vi "Homework 1.vi"() -> ()   [LabVIEW 2018]
uses:
  Control 1.ctl
  <vilib>/DAQmx/write.llb/DAQmx Write (Digital Bool 1Line 1Point).vi
  <vilib>/DAQmx/read.llb/DAQmx Read (Analog DBL 1Chan 1Samp).vi
  <vilib>/DAQmx/create/channels.llb/DAQmx Create Channel (DO-Digital Output).vi
  <vilib>/DAQmx/miscellaneous.llb/DAQmx Fill In Error Info.vi
  <vilib>/DAQmx/create/channels.llb/DAQmx Create Channel (AI-Voltage-Basic).vi
panel:
  out "Image Out":T1(plugin-control)
  in  "Izbor predmeta":enum16{"Predmet A", "Predmet B", "Predmet C"}(ring)
  in  "a":bool
  in  "Promeni predmet":bool
  in  "Ukloni alarm":bool
  in  "Pokreni traku":bool
  in  "Predmet je na traci":bool
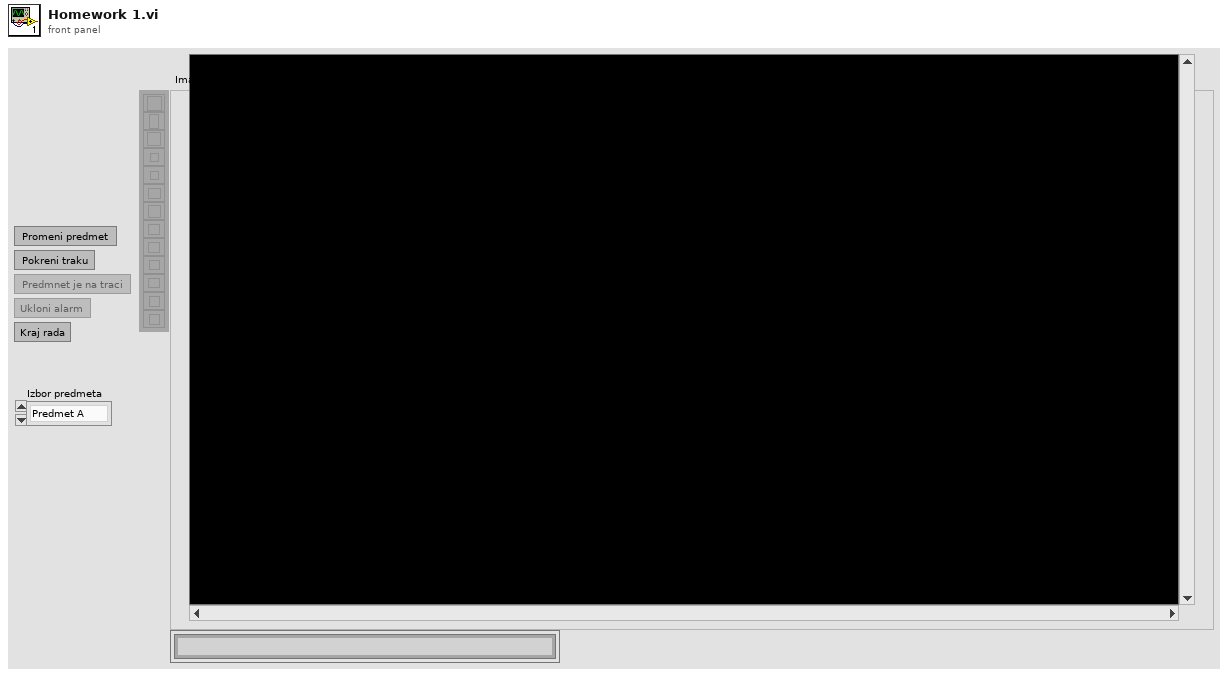
[diagram p1: front panel]
types:
  T1 = typedef "IMAQ Image.ctl" = refnum<image>
  T2 = enum16{"open", "replace", "create", "open or create", "replace or create", "replace or create with confirmation"}
  T3 = typedef "Control 1.ctl" = enum16{"IzbPr", "PrTrk", "Alarm", "Kretanje", "Slikanje"}
  T4 = enum8{"Enabled", "Disabled", "Disabled and Grayed Out"}
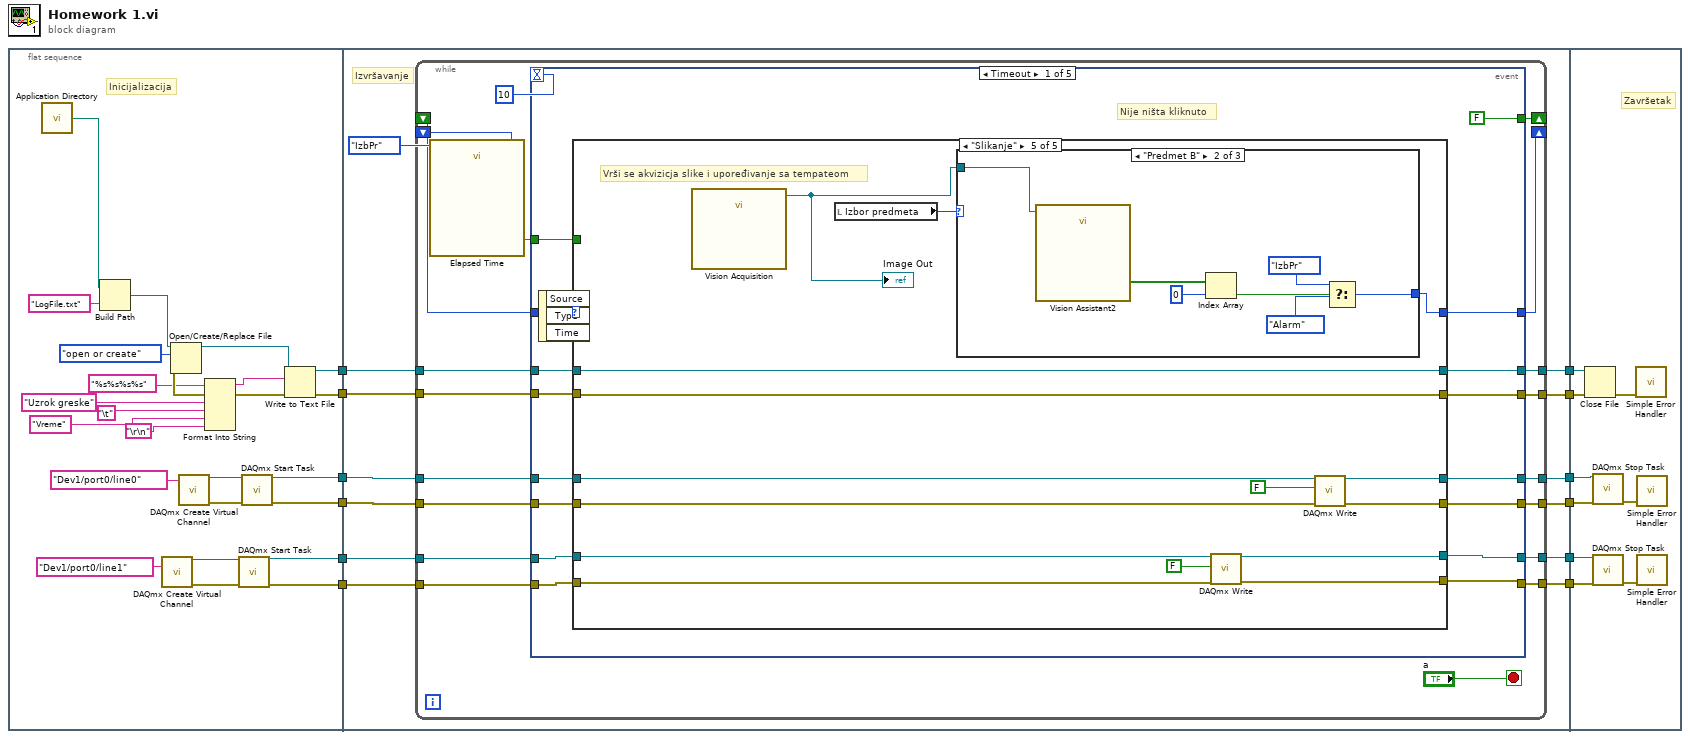
[diagram p0: block diagram]
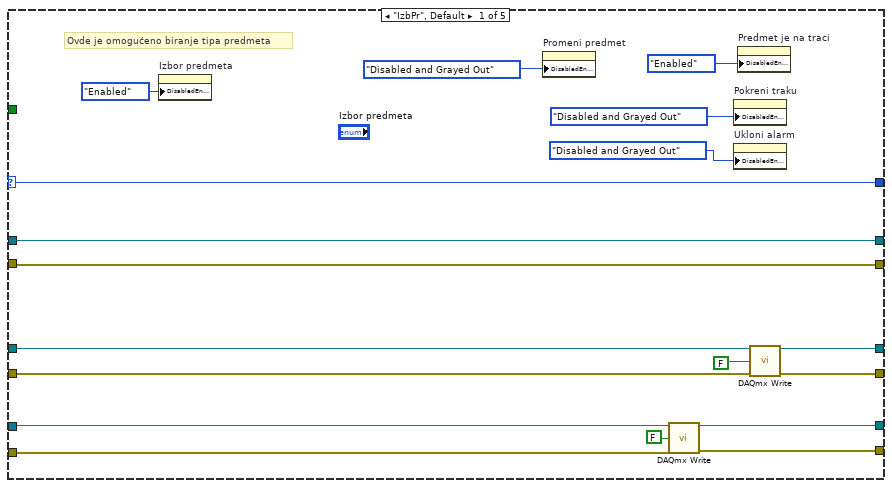
[diagram p2: hidden frame]
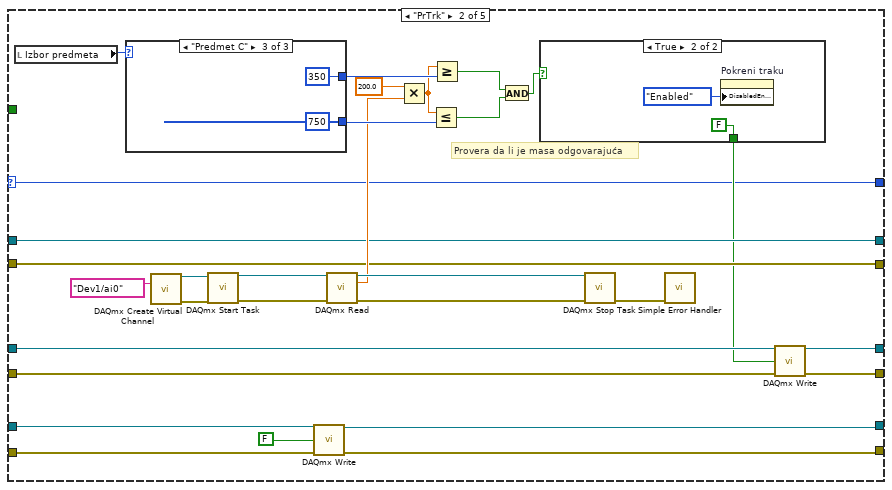
[diagram p3: hidden frame]
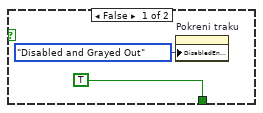
[diagram p4: hidden frame]
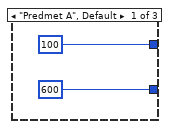
[diagram p5: hidden frame]
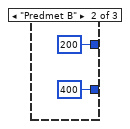
[diagram p6: hidden frame]
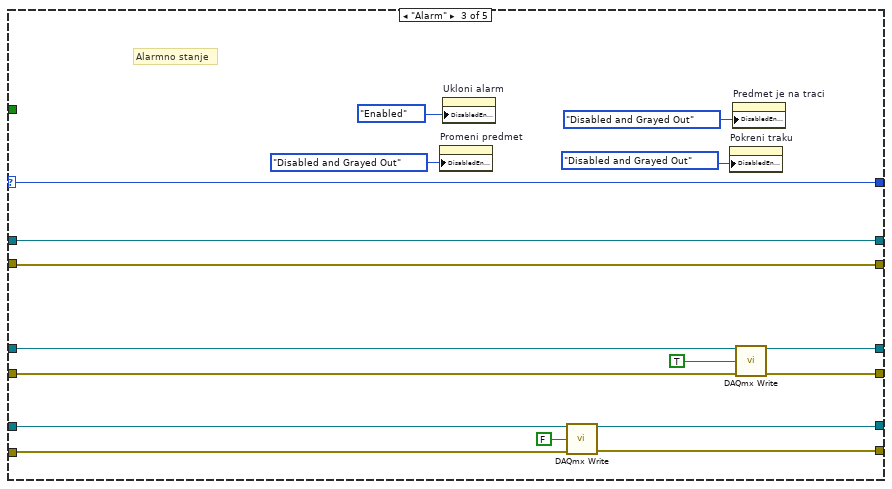
[diagram p7: hidden frame]
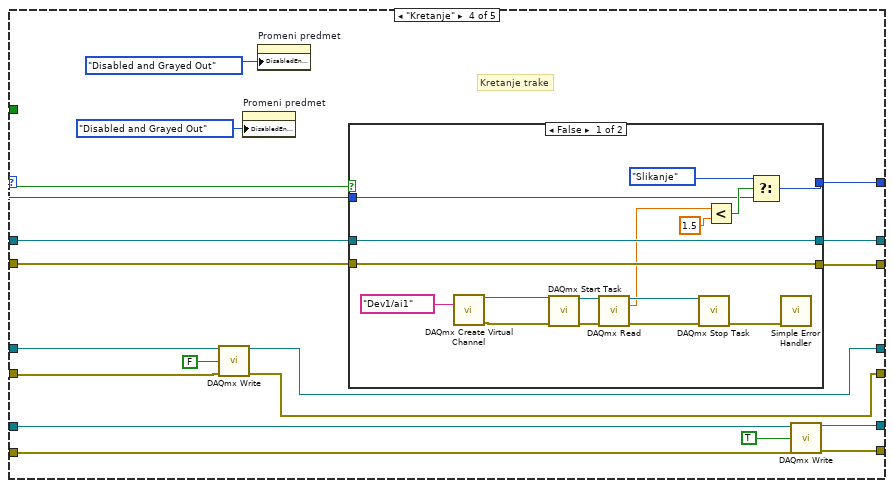
[diagram p8: hidden frame]
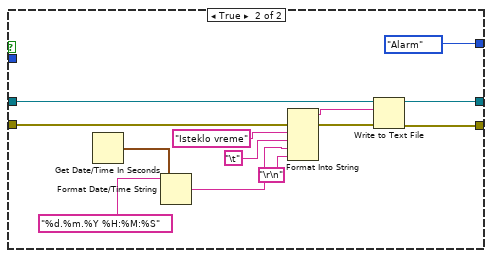
[diagram p9: hidden frame]
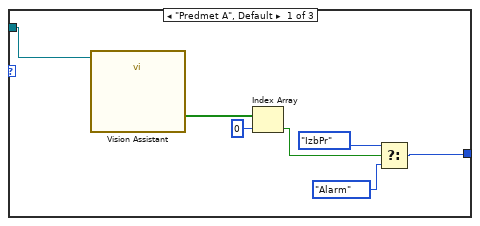
[diagram p10: hidden frame]
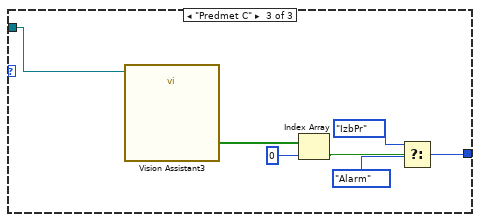
[diagram p11: hidden frame]
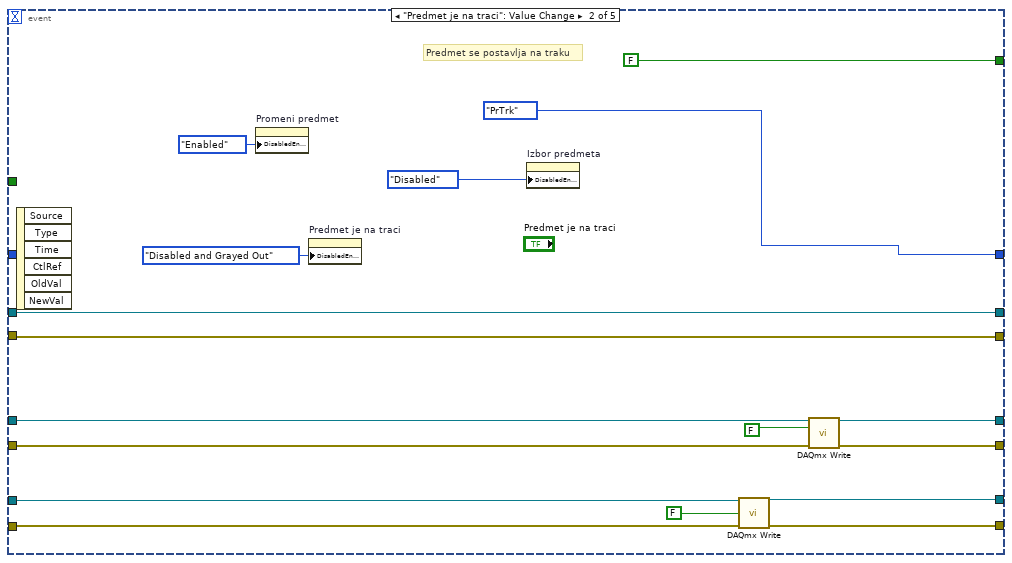
[diagram p12: hidden frame]
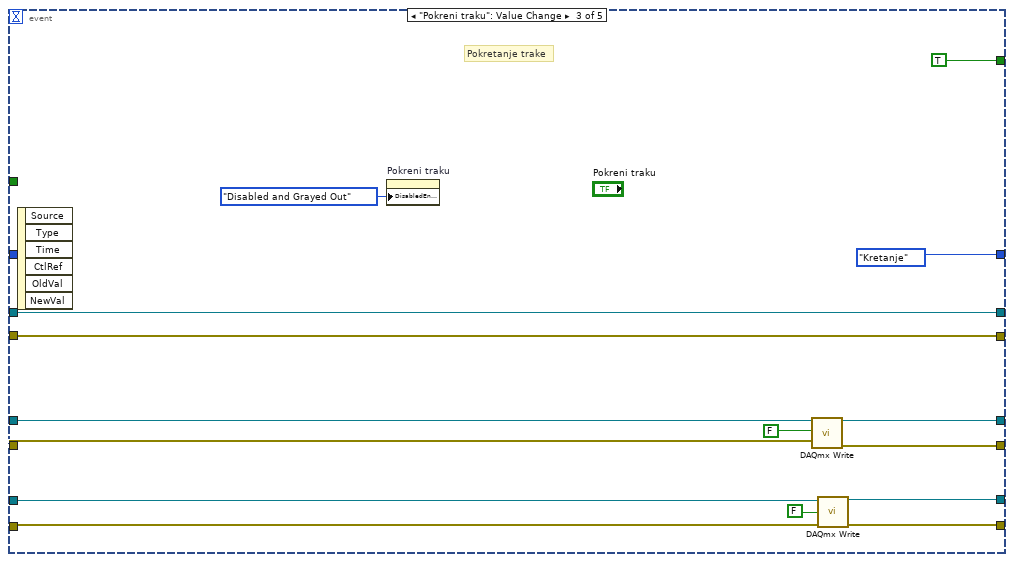
[diagram p13: hidden frame]
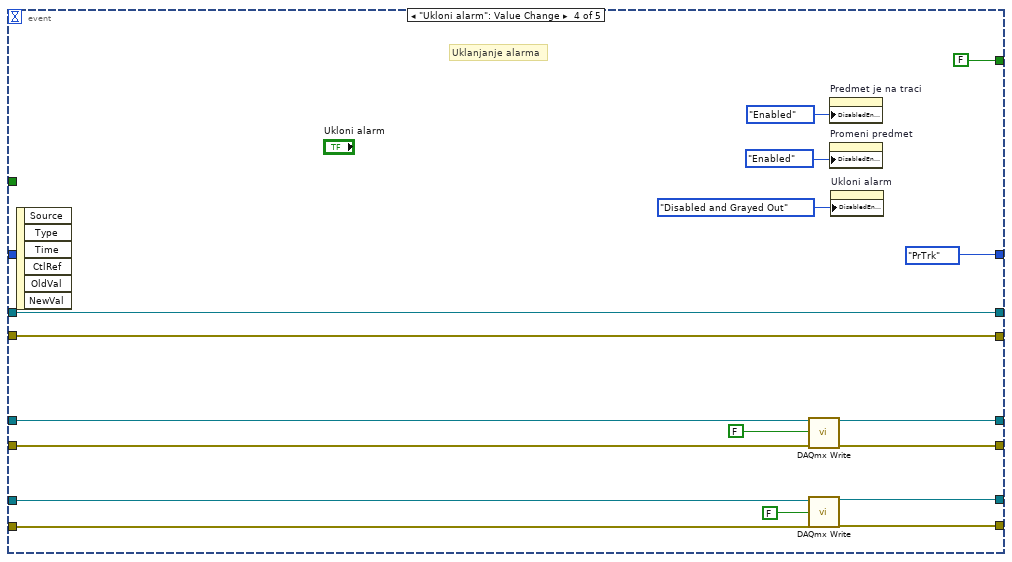
[diagram p14: hidden frame]
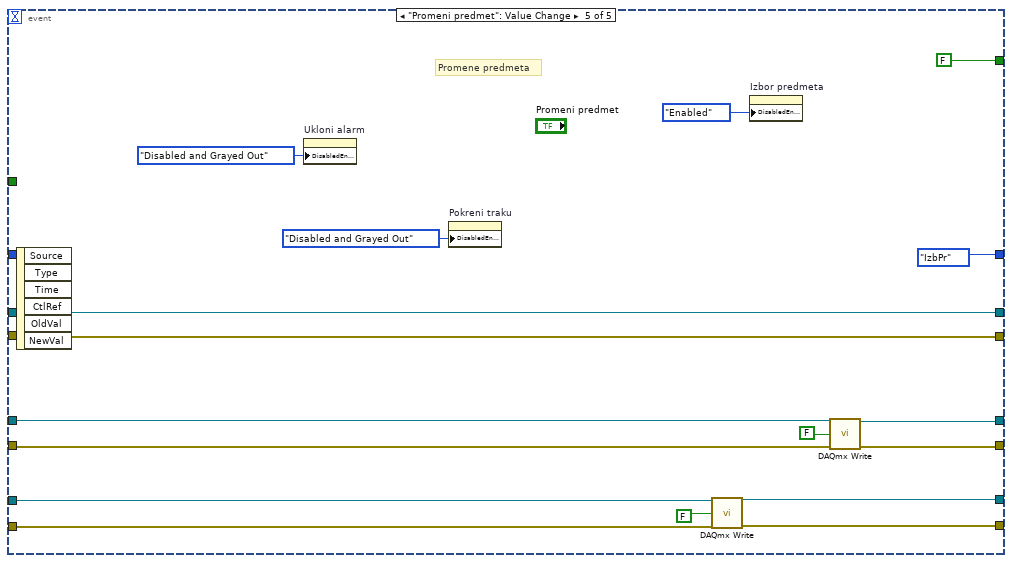
[diagram p15: hidden frame]
diagram:
  n1 = flat-sequence {
    tunnel: [w21] -> w12
    tunnel: [w20] -> w11
    tunnel: [w16] -> w6
    tunnel: [w15] -> w5
    tunnel: [w13] -> w2
    tunnel: [w14] -> w1
    tunnel: w12 -> [w50]
    tunnel: w11 -> [w49]
    tunnel: [w48] -> w10
    tunnel: [w47] -> w9
    tunnel: [w45] -> w8
    tunnel: [w44] -> w7
    tunnel: w6 -> [w43]
    tunnel: w5 -> [w42]
    tunnel: [w41] -> w4
    tunnel: [w40] -> w3
    tunnel: w2 -> [w38]
    tunnel: w1 -> [w39]
    tunnel: w10 -> [w318]
    tunnel: w9 -> [w317]
    tunnel: w8 -> [w316]
    tunnel: w7 -> [w315]
    tunnel: w4 -> [w312]
    tunnel: w3 -> [w311]
    frame #0 {
      # "Inicijalizacija"
      n2 = call <vilib>:"Application Directory.vi"() -> ("Application Directory"=w34:path)
      n3 = Build Path(base path=w34, name or relative path="LogFile.txt") -> (appended path=w36:path)
      n4 = call-poly <vilib>:"DAQmx Create Virtual Channel.vi"("lines"=tag "Dev1/port0/line1") -> ("task out"=w19:refnum<k21>, "error out"=w18:errorcluster)  [unwired: 13 in]
      n5 = Open/Create/Replace File(file path (use dialog)=w36, operation (0:open)=T2."open or create") -> (refnum out=w33:refnum<file>, error out=w31:errorcluster)  [unwired: 4 in, 1 out]
      n6 = call-poly <vilib>:"DAQmx Create Virtual Channel.vi"("lines"=tag "Dev1/port0/line0") -> ("task out"=w24:refnum<k21>, "error out"=w23:errorcluster)  [unwired: 13 in]
      n7 = Format Into String(format string="%s%s%s%s" ("prompt (Choose or enter file path)"), error in=w31, "Uzrok greske" ("input 1"), "\t", "Vreme" ("input 3"), "\r\n") -> (resulting string=w32:string, error out=w30:errorcluster)  [unwired: 1 in]
      n8 = call <vilib>:"DAQmx Start Task.vi"("task/channels in"=w19, "error in"=w18) -> ("task out"=w16:refnum<k21>, "error out"=w15:errorcluster)  [unwired: 12 in]
      n9 = call <vilib>:"DAQmx Start Task.vi"("task/channels in"=w24, "error in"=w23) -> ("task out"=w21:refnum<k21>, "error out"=w20:errorcluster)  [unwired: 12 in]
      n10 = Write to Text File(file (use dialog)=w33, text=w32, error in=w30) -> (refnum out=w14:refnum<file>, error out=w13:errorcluster)  [unwired: 1 in, 1 out]
    }
    frame #1 {
      # "Izvršavanje"
      n11 = while {
        shift-right: [w69] -> _
        shift-left: Control_1."IzbPr" ("Enum") -> [w68]
        tunnel: w50 -> [w67]
        tunnel: w49 -> [w66]
        tunnel: [w65] -> w48
        tunnel: [w64] -> w47
        shift-right: [w63] -> _
        shift-left: _ -> [w62]
        tunnel: [w59] -> w45
        tunnel: [w51] -> w44
        tunnel: w43 -> [w58]
        tunnel: w42 -> [w57]
        tunnel: [w56] -> w41
        tunnel: [w55] -> w40
        tunnel: w39 -> [w54]
        tunnel: w38 -> [w53]
        stop <- "a" stop-if-true
        n12 = call "Elapsed Time"("Reset"=w62) -> ("Time has Elapsed"=w61:bool)  [unwired: 11 in, 7 out]
        n13 = event shown="[0] Timeout" {
          selector: _ -> [_ _ _ _ _]
          dyn-events: _ -> [_ _ _ _ _]
          timeout: 10 -> [_ _ _ _ _]
          tunnel: [w85 Control_1."PrTrk" ("Enum") Control_1."Kretanje" ("Enum") Control_1."PrTrk" ("Enum") Control_1."IzbPr" ("Enum")] -> w69
          tunnel: w68 -> [w84 _ _ _ _]
          tunnel: w67 -> [w83 w256 w274 w291 w309]
          tunnel: w66 -> [w82 w257 w273 w277 w301]
          tunnel: [w81 w259 w276 w290 w296] -> w65
          tunnel: [w80 w258 w275 w289 w308] -> w64
          tunnel: [FALSE FALSE TRUE FALSE FALSE] -> w63
          tunnel: w61 -> [w78 _ _ _ _]
          tunnel: [w76 w252 w269 w287 w305] -> w59
          tunnel: [w75 w251 w268 w286 w304] -> w51
          tunnel: w58 -> [w77 w250 w267 w285 w303]
          tunnel: w57 -> [w74 w249 w266 w284 w302]
          tunnel: [w73 w248 w265 w281 w298] -> w56
          tunnel: [w72 w247 w264 w280 w297] -> w55
          tunnel: w54 -> [w71 w248 w265 w281 w298]
          tunnel: w53 -> [w70 w247 w264 w280 w297]
          event Timeout {
            # "Nije ništa kliknuto"
            n14 = event-data() -> ()  [unwired: 1 in, 3 out]
            n15 = case shown="\"Slikanje\"" w84 {
              selector: w84 -> [w103 w104 w157 w176 _]
              tunnel: [w103 w104 w157 w161 w217] -> w85
              tunnel: w83 -> [w100 w132 w155 w178 w223]
              tunnel: w82 -> [w93 w117 w154 w171 w221]
              tunnel: [w99 w131 w153 w173 w222] -> w81
              tunnel: [w98 w130 w152 w172 w220] -> w80
              tunnel: w78 -> [_ _ _ w174 _]
              tunnel: w77 -> [w90 w114 w147 w170 w214]
              tunnel: [w92 w112 w150 w169 w212] -> w76
              tunnel: [w91 w111 w149 w168 w211] -> w75
              tunnel: w74 -> [w89 w113 w146 w167 w213]
              tunnel: [w88 w109 w145 w165 w210] -> w73
              tunnel: [w87 w110 w144 w164 w209] -> w72
              tunnel: w71 -> [w88 w109 w145 w163 w210]
              tunnel: w70 -> [w87 w110 w144 w162 w209]
              frame "IzbPr", Default {
                # "Ovde je omogućeno biranje tipa predmeta"
                n16 = property on="Izbor predmeta" class="Enum (strict)"("DisabledEnum"=T4."Enabled" ("Disabled")) -> ()  [unwired: 2 in, 2 out]
                n17 = property on="Promeni predmet" class="Bool"("DisabledEnum"=T4."Disabled and Grayed Out" ("Disabled")) -> ()  [unwired: 2 in, 2 out]
                n18 = call-poly <vilib>:"DAQmx Write.vi"("task/channels in"=w90, "data"=FALSE, "error in"=w89) -> ("task out"=w92:refnum<k21>, "error out"=w91:errorcluster)  [unwired: 10 in, 1 out]
                n19 = property on="Pokreni traku" class="Bool"("DisabledEnum"=T4."Disabled and Grayed Out" ("Disabled")) -> ()  [unwired: 2 in, 2 out]
                n20 = property on="Ukloni alarm" class="Bool"("DisabledEnum"=T4."Disabled and Grayed Out" ("Disabled")) -> ()  [unwired: 2 in, 2 out]
                n21 = property on="Predmet je na traci" class="Bool"("DisabledEnum"=T4."Enabled" ("Disabled")) -> ()  [unwired: 2 in, 2 out]
                n22 = call-poly <vilib>:"DAQmx Write.vi"("task/channels in"=w100, "data"=FALSE, "error in"=w93) -> ("task out"=w99:refnum<k21>, "error out"=w98:errorcluster)  [unwired: 10 in, 1 out]
              }
              frame "PrTrk" {
                # "Provera da li je masa odgovarajuća"
                n23 = local read "Izbor predmeta"() -> (w115:enum16{"Predmet A", "Predmet B", "Predmet C"})
                n24 = case shown="\"Predmet C\"" w115 {
                  tunnel: [100 200 350] -> w133
                  tunnel: [600 400 750] -> w123
                  frame "Predmet A", Default {
                  }
                  frame "Predmet B" {
                  }
                  frame "Predmet C" {
                  }
                }
                n25 = call-poly <vilib>:"DAQmx Create Virtual Channel.vi"("physical channels"=tag "Dev1/ai0") -> ("task out"=w126:refnum<k21>, "error out"=w127:errorcluster)  [unwired: 13 in]
                n26 = call <vilib>:"DAQmx Start Task.vi"("task/channels in"=w126, "error in"=w127) -> ("task out"=w124:refnum<k21>, "error out"=w119:errorcluster)  [unwired: 12 in]
                n27 = call-poly <vilib>:"DAQmx Write.vi"("task/channels in"=w114, "data"=FALSE, "error in"=w113) -> ("task out"=w112:refnum<k21>, "error out"=w111:errorcluster)  [unwired: 10 in, 1 out]
                n28 = call-poly <vilib>:"DAQmx Read.vi"("task/channels in"=w124, "error in"=w119) -> ("task out"=w122:refnum<k21>, "data"=w116:dbl, "error out"=w121:errorcluster)  [unwired: 11 in]
                n29 = Multiply(x=200.0 ("y"), y=w116) -> (x*y=w107:dbl)
                n30 = Less Or Equal?(x=w107, y=w123) -> (x <= y?=w105:bool)
                n31 = Greater Or Equal?(x=w107, y=w133) -> (x >= y?=w106:bool)
                n32 = And(x=w106, y=w105) -> (x .and. y?=w118:bool)
                n33 = case shown="True" w118 {
                  tunnel: [TRUE FALSE] -> w108
                  frame False {
                    n34 = property on="Pokreni traku" class="Bool"("DisabledEnum"=T4."Disabled and Grayed Out" ("Disabled")) -> ()  [unwired: 2 in, 2 out]
                  }
                  frame True {
                    n35 = property on="Pokreni traku" class="Bool"("DisabledEnum"=T4."Enabled" ("Disabled")) -> ()  [unwired: 2 in, 2 out]
                  }
                }
                n36 = call <vilib>:"DAQmx Stop Task.vi"("task/channels in"=w122, "error in"=w121) -> ("error out"=w128:errorcluster)  [unwired: 12 in, 1 out]
                n37 = call <vilib>:"Simple Error Handler.vi"("error in (no error)"=w128) -> ()  [unwired: 4 in, 5 out]
                n38 = call-poly <vilib>:"DAQmx Write.vi"("task/channels in"=w132, "data"=w108, "error in"=w117) -> ("task out"=w131:refnum<k21>, "error out"=w130:errorcluster)  [unwired: 10 in, 1 out]
              }
              frame "Alarm" {
                # "Alarmno stanje"
                n39 = property on="Promeni predmet" class="Bool"("DisabledEnum"=T4."Disabled and Grayed Out" ("Disabled")) -> ()  [unwired: 2 in, 2 out]
                n40 = property on="Ukloni alarm" class="Bool"("DisabledEnum"=T4."Enabled" ("Disabled")) -> ()  [unwired: 2 in, 2 out]
                n41 = call-poly <vilib>:"DAQmx Write.vi"("task/channels in"=w147, "data"=FALSE, "error in"=w146) -> ("task out"=w150:refnum<k21>, "error out"=w149:errorcluster)  [unwired: 10 in, 1 out]
                n42 = property on="Pokreni traku" class="Bool"("DisabledEnum"=T4."Disabled and Grayed Out" ("Disabled")) -> ()  [unwired: 2 in, 2 out]
                n43 = property on="Predmet je na traci" class="Bool"("DisabledEnum"=T4."Disabled and Grayed Out" ("Disabled")) -> ()  [unwired: 2 in, 2 out]
                n44 = call-poly <vilib>:"DAQmx Write.vi"("task/channels in"=w155, "data"=TRUE, "error in"=w154) -> ("task out"=w153:refnum<k21>, "error out"=w152:errorcluster)  [unwired: 10 in, 1 out]
              }
              frame "Kretanje" {
                # "Kretanje trake"
                n45 = call-poly <vilib>:"DAQmx Write.vi"("task/channels in"=w178, "data"=FALSE, "error in"=w171) -> ("task out"=w173:refnum<k21>, "error out"=w172:errorcluster)  [unwired: 10 in, 1 out]
                n46 = property on="Promeni predmet" class="Bool"("DisabledEnum"=T4."Disabled and Grayed Out" ("Disabled")) -> ()  [unwired: 2 in, 2 out]
                n47 = property on="Promeni predmet" class="Bool"("DisabledEnum"=T4."Disabled and Grayed Out" ("Disabled")) -> ()  [unwired: 2 in, 2 out]
                n48 = case shown="False" w174 {
                  tunnel: w176 -> [w187 _]
                  tunnel: [w184 w204] -> w165
                  tunnel: [w183 w203] -> w164
                  tunnel: w162 -> [w183 w198]
                  tunnel: w163 -> [w184 w197]
                  tunnel: [w182 Control_1."Alarm" ("Enum")] -> w161
                  frame False {
                    n49 = call-poly <vilib>:"DAQmx Create Virtual Channel.vi"("physical channels"=tag "Dev1/ai1") -> ("task out"=w195:refnum<k21>, "error out"=w194:errorcluster)  [unwired: 13 in]
                    n50 = call <vilib>:"DAQmx Start Task.vi"("task/channels in"=w195, "error in"=w194) -> ("task out"=w190:refnum<k21>, "error out"=w189:errorcluster)  [unwired: 12 in]
                    n51 = call-poly <vilib>:"DAQmx Read.vi"("task/channels in"=w190, "error in"=w189) -> ("task out"=w185:refnum<k21>, "data"=w180:dbl, "error out"=w191:errorcluster)  [unwired: 11 in]
                    n52 = call <vilib>:"DAQmx Stop Task.vi"("task/channels in"=w185, "error in"=w191) -> ("error out"=w192:errorcluster)  [unwired: 12 in, 1 out]
                    n53 = Less?(x=w180, y=1.5) -> (x < y?=w188:bool)
                    n54 = Select(t=Control_1."Slikanje" ("Enum"), s=w188, f=w187) -> (s? t:f=w182:T3)
                    n55 = call <vilib>:"Simple Error Handler.vi"("error in (no error)"=w192) -> ()  [unwired: 4 in, 5 out]
                  }
                  frame True {
                    n56 = Get Date/Time In Seconds() -> (seconds since 1Jan1904=w206:timestamp)
                    n57 = Format Date/Time String(time format string (%c)="%d.%m.%Y %H:%M:%S", seconds (now)=w206) -> (date/time string=w200:string)  [unwired: 1 in]
                    n58 = Format Into String(error in=w198, "Isteklo vreme" ("input 1"), "\t", w200, "\r\n") -> (resulting string=w207:string, error out=w202:errorcluster)  [unwired: 2 in]
                    n59 = Write to Text File(file (use dialog)=w197, text=w207, error in=w202) -> (refnum out=w204:refnum<file>, error out=w203:errorcluster)  [unwired: 1 in, 1 out]
                  }
                }
                n60 = call-poly <vilib>:"DAQmx Write.vi"("task/channels in"=w170, "data"=TRUE, "error in"=w167) -> ("task out"=w169:refnum<k21>, "error out"=w168:errorcluster)  [unwired: 10 in, 1 out]
              }
              frame "Slikanje" {
                # "Vrši se akvizicja slike i upoređivanje sa tempateom"
                n61 = call "Vision Acquisition"() -> ("Image Out"=w215:T1)  [unwired: 25 in, 2 out]
                "Image Out" <- w215
                n62 = local read "Izbor predmeta"() -> (w216:enum16{"Predmet A", "Predmet B", "Predmet C"})
                n63 = case shown="\"Predmet B\"" w216 {
                  tunnel: w215 -> [w230 w234 w241]
                  tunnel: [w225 w232 w238] -> w217
                  frame "Predmet A", Default {
                    n64 = call "Vision Assistant"("Image In"=w230) -> ("Match Flag (Color Matching 1)"=w229:bool[])  [unwired: 24 in, 2 out]
                    n65 = Index Array(array=w229, index=0) -> (element=w226:bool)
                    n66 = Select(t=Control_1."IzbPr" ("Enum"), s=w226, f=Control_1."Alarm" ("Enum")) -> (s? t:f=w225:T3)
                  }
                  frame "Predmet B" {
                    n67 = call "Vision Assistant2"("Image In"=w234) -> ("Match Flag (Color Matching 1)"=w231:bool[])  [unwired: 24 in, 2 out]
                    n68 = Index Array(array=w231, index=0) -> (element=w233:bool)
                    n69 = Select(t=Control_1."IzbPr" ("Enum"), s=w233, f=Control_1."Alarm" ("Enum")) -> (s? t:f=w232:T3)
                  }
                  frame "Predmet C" {
                    n70 = call "Vision Assistant3"("Image In"=w241) -> ("Match Flag (Color Matching 1)"=w239:bool[])  [unwired: 24 in, 2 out]
                    n71 = Index Array(array=w239, index=0) -> (element=w240:bool)
                    n72 = Select(t=Control_1."IzbPr" ("Enum"), s=w240, f=Control_1."Alarm" ("Enum")) -> (s? t:f=w238:T3)
                  }
                }
                n73 = call-poly <vilib>:"DAQmx Write.vi"("task/channels in"=w214, "data"=FALSE, "error in"=w213) -> ("task out"=w212:refnum<k21>, "error out"=w211:errorcluster)  [unwired: 10 in, 1 out]
                n74 = call-poly <vilib>:"DAQmx Write.vi"("task/channels in"=w223, "data"=FALSE, "error in"=w221) -> ("task out"=w222:refnum<k21>, "error out"=w220:errorcluster)  [unwired: 10 in, 1 out]
              }
            }
          }
          event "Predmet je na traci": Value Change {
            # "Predmet se postavlja na traku"
            n75 = event-data() -> ()  [unwired: 1 in, 6 out]
            n76 = property on="Promeni predmet" class="Bool"("DisabledEnum"=T4."Enabled" ("Disabled")) -> ()  [unwired: 2 in, 2 out]
            n77 = property on="Predmet je na traci" class="Bool"("DisabledEnum"=T4."Disabled and Grayed Out" ("Disabled")) -> ()  [unwired: 2 in, 2 out]
            n78 = property on="Izbor predmeta" class="Enum (strict)"("DisabledEnum"=T4."Disabled" ("Disabled")) -> ()  [unwired: 2 in, 2 out]
            n79 = call-poly <vilib>:"DAQmx Write.vi"("task/channels in"=w250, "data"=FALSE, "error in"=w249) -> ("task out"=w252:refnum<k21>, "error out"=w251:errorcluster)  [unwired: 10 in, 1 out]
            n80 = call-poly <vilib>:"DAQmx Write.vi"("task/channels in"=w256, "data"=FALSE, "error in"=w257) -> ("task out"=w259:refnum<k21>, "error out"=w258:errorcluster)  [unwired: 10 in, 1 out]
          }
          event "Pokreni traku": Value Change {
            # "Pokretanje trake"
            n81 = event-data() -> ()  [unwired: 1 in, 6 out]
            n82 = property on="Pokreni traku" class="Bool"("DisabledEnum"=T4."Disabled and Grayed Out" ("Disabled")) -> ()  [unwired: 2 in, 2 out]
            n83 = call-poly <vilib>:"DAQmx Write.vi"("task/channels in"=w274, "data"=FALSE, "error in"=w273) -> ("task out"=w276:refnum<k21>, "error out"=w275:errorcluster)  [unwired: 10 in, 1 out]
            n84 = call-poly <vilib>:"DAQmx Write.vi"("task/channels in"=w267, "data"=FALSE, "error in"=w266) -> ("task out"=w269:refnum<k21>, "error out"=w268:errorcluster)  [unwired: 10 in, 1 out]
          }
          event "Ukloni alarm": Value Change {
            # "Uklanjanje alarma"
            n85 = event-data() -> ()  [unwired: 1 in, 6 out]
            n86 = call-poly <vilib>:"DAQmx Write.vi"("task/channels in"=w291, "data"=FALSE, "error in"=w277) -> ("task out"=w290:refnum<k21>, "error out"=w289:errorcluster)  [unwired: 10 in, 1 out]
            n87 = call-poly <vilib>:"DAQmx Write.vi"("task/channels in"=w285, "data"=FALSE, "error in"=w284) -> ("task out"=w287:refnum<k21>, "error out"=w286:errorcluster)  [unwired: 10 in, 1 out]
            n88 = property on="Predmet je na traci" class="Bool"("DisabledEnum"=T4."Enabled" ("Disabled")) -> ()  [unwired: 2 in, 2 out]
            n89 = property on="Promeni predmet" class="Bool"("DisabledEnum"=T4."Enabled" ("Disabled")) -> ()  [unwired: 2 in, 2 out]
            n90 = property on="Ukloni alarm" class="Bool"("DisabledEnum"=T4."Disabled and Grayed Out" ("Disabled")) -> ()  [unwired: 2 in, 2 out]
          }
          event "Promeni predmet": Value Change {
            # "Promene predmeta"
            n91 = event-data() -> ()  [unwired: 1 in, 6 out]
            n92 = property on="Ukloni alarm" class="Bool"("DisabledEnum"=T4."Disabled and Grayed Out" ("Disabled")) -> ()  [unwired: 2 in, 2 out]
            n93 = property on="Pokreni traku" class="Bool"("DisabledEnum"=T4."Disabled and Grayed Out" ("Disabled")) -> ()  [unwired: 2 in, 2 out]
            n94 = call-poly <vilib>:"DAQmx Write.vi"("task/channels in"=w303, "data"=FALSE, "error in"=w302) -> ("task out"=w305:refnum<k21>, "error out"=w304:errorcluster)  [unwired: 10 in, 1 out]
            n95 = property on="Izbor predmeta" class="Enum (strict)"("DisabledEnum"=T4."Enabled" ("Disabled")) -> ()  [unwired: 2 in, 2 out]
            n96 = call-poly <vilib>:"DAQmx Write.vi"("task/channels in"=w309, "data"=FALSE, "error in"=w301) -> ("task out"=w296:refnum<k21>, "error out"=w308:errorcluster)  [unwired: 10 in, 1 out]
          }
        }
      }
    }
    frame #2 {
      # "Završetak"
      n97 = Close File(refnum=w312, error in=w311) -> (error out=w319:errorcluster)  [unwired: 1 out]
      n98 = call <vilib>:"DAQmx Stop Task.vi"("task/channels in"=w318, "error in"=w317) -> ("error out"=w314:errorcluster)  [unwired: 12 in, 1 out]
      n99 = call <vilib>:"DAQmx Stop Task.vi"("task/channels in"=w316, "error in"=w315) -> ("error out"=w313:errorcluster)  [unwired: 12 in, 1 out]
      n100 = call <vilib>:"Simple Error Handler.vi"("error in (no error)"=w319) -> ()  [unwired: 4 in, 5 out]
      n101 = call <vilib>:"Simple Error Handler.vi"("error in (no error)"=w314) -> ()  [unwired: 4 in, 5 out]
      n102 = call <vilib>:"Simple Error Handler.vi"("error in (no error)"=w313) -> ()  [unwired: 4 in, 5 out]
    }
  }
